vi "Load Offline Map.vi"() -> ()   [LabVIEW 2014]
uses:
  C:/Robotic_Systems/Products/Surveyor/Software/Ground Station/Data/Mapping DLL/GMap.NET.WindowsForms.dll
  Data/Mapping DLL/GMap.NET.WindowsForms.dll
  <vilib>/Utility/miscctls.llb/LVPoint32TypeDef.ctl
  <vilib>/Utility/miscctls.llb/LVPositionTypeDef.ctl
  C:/Robotic_Systems/Products/Surveyor/Software/Ground Station/Data/Mapping DLL/GMap.NET.Core.dll
  Data/Mapping DLL/GMap.NET.Core.dll
  System.Drawing
  System.Windows.Forms
panel:
  in  "Position":T1
  in  "reference out":refnum<k24>
  out "Coords":T2
  out "Lng":dbl format="%#.7g"
  out "Lat":dbl format="%#.7g"
  out "Y":i32
  out "X":i32
  out "Name":string
  out "Case Test":bool
  out "ImportFromGMDB":bool
  in  "Home Button":bool
  out "Center Map Long":dbl format="%#.7g"
  out "Center Map Lat":dbl format="%#.7g"
  out "Current Zoom":dbl
  in  "stop Program":bool
  in  "Offline Map file path (.gmdb)":path
  in  "Map Mode":i32(ring)=2 items=["ServerOnly", "ServerAndCache", "CacheOnly"]
  in  "GMapControl":refnum<k24>(container)
  # "How to Use Map\n\nDragging: hold down right mouse button and move mouse\nZoom: Use mouse scroll Wheel"
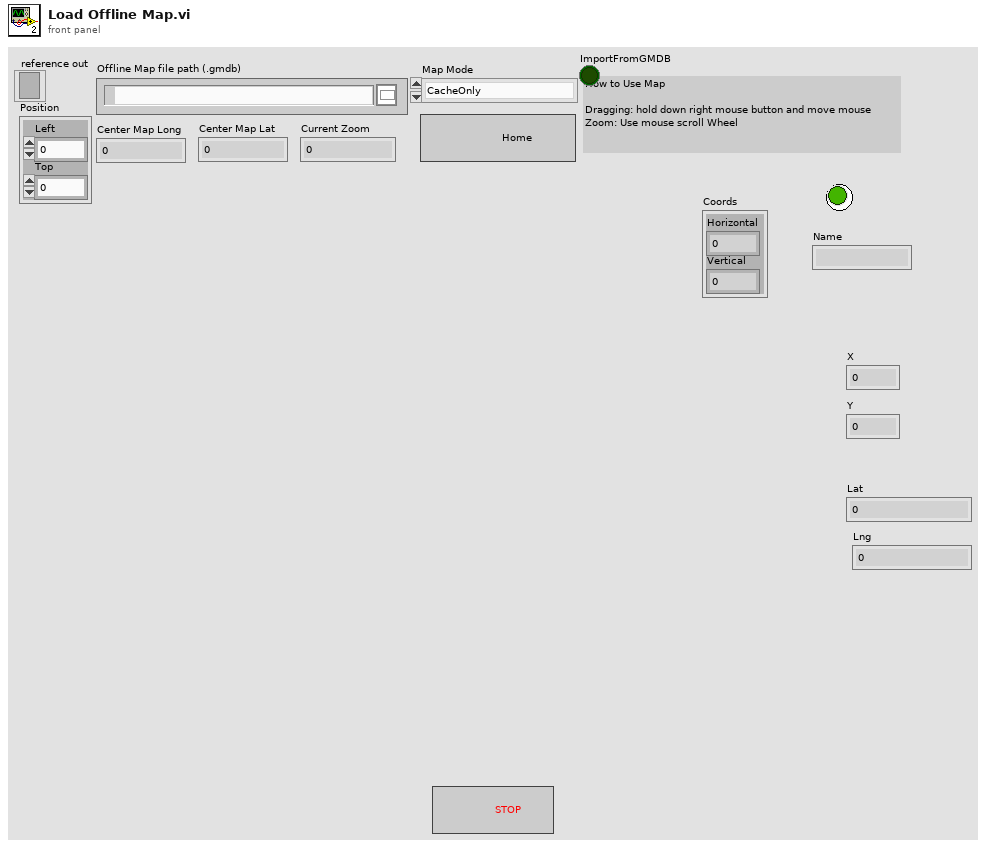
[diagram p1: front panel]
types:
  T1 = typedef "LVPositionTypeDef.ctl" = cluster{"Left":i32, "Top":i32}
  T2 = typedef "LVPoint32TypeDef.ctl" = cluster{"Horizontal":i32, "Vertical":i32}
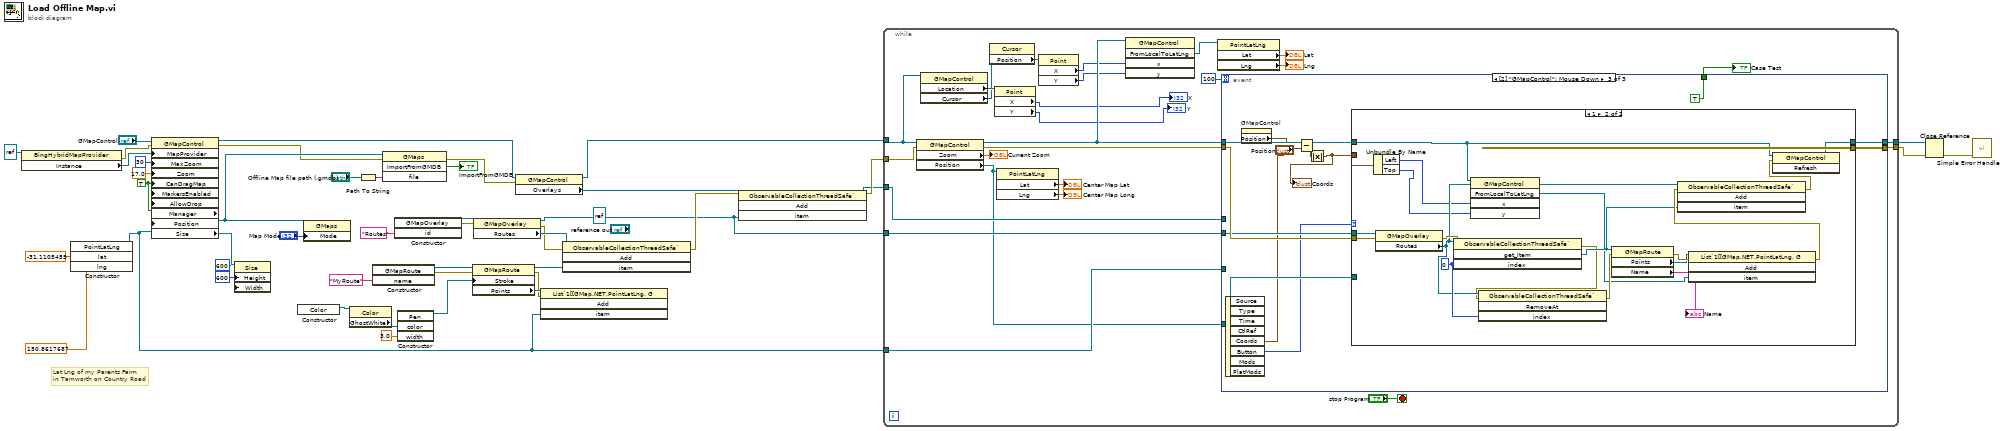
[diagram p0: block diagram]
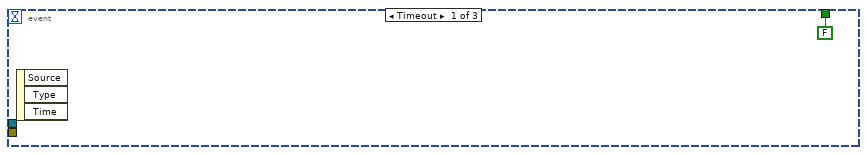
[diagram p2: hidden frame]
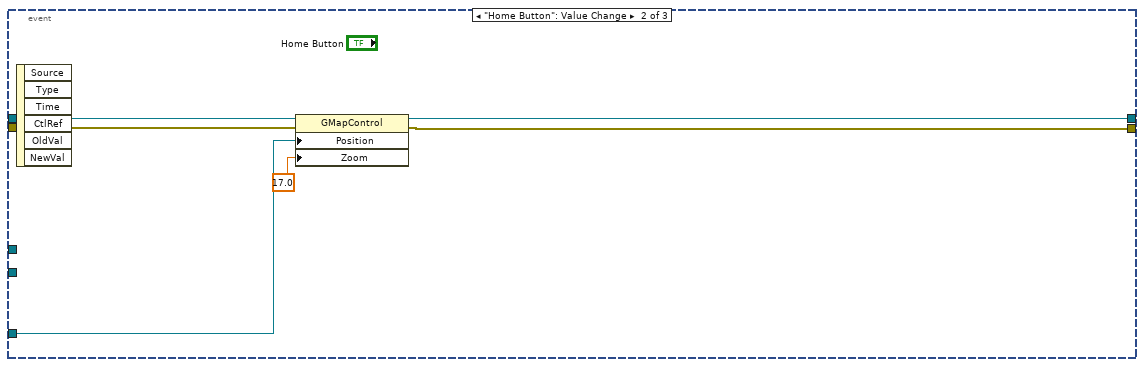
[diagram p3: hidden frame]
diagram:
  (unwired) refnum<k24> refnum ("reference out")
  w41 = TRUE ("CanDragMap")
  # "Lat Lng of my Parents Farm\nin Tamworth on Country Road"
  n1 = property class="BingHybridMapProvider"(reference=refnum<k24> refnum) -> (error out=w33:errorcluster, "Instance"=w43:refnum<k24>)  [unwired: 1 in, 1 out]
  n2 = constructor class="PointLatLng"("lat"=-31.1105459, "lng"=150.8617687) -> (reference out=w9:refnum<k24>)  [unwired: 3 in, 4 out]
  n3 = property class="GMapControl"(reference="GMapControl", error in=w33, "MapProvider"=w43, "MaxZoom"=30, "Zoom"=17.0, "CanDragMap"=w41, "MarkersEnabled"=w41, "AllowDrop"=w41, "Position"=w9) -> (reference out=w24:refnum<k24>, error out=w32:errorcluster, "Manager"=w36:refnum<k24>, "Size"=w3:refnum<k24>)
  n4 = property class="Size"(reference=w3, "Height"=600, "Width"=600) -> ()  [unwired: 1 in, 2 out]
  n5 = constructor class="Color"() -> (reference out=w18:refnum<k24>)  [unwired: 3 in, 2 out]
  n6 = property class="GMaps"(reference=w36, "Mode"="Map Mode") -> ()  [unwired: 1 in, 2 out]
  n7 = property class="Color"(reference=w18) -> ("GhostWhite"=w21:refnum<k24>)  [unwired: 1 in, 2 out]
  n8 = Path To String(path="Offline Map file path (.gmdb)") -> (string=w35:string)
  n9 = constructor class="GMapRoute"("name"="MyRoute") -> (reference out=w5:refnum<k24>, error out=w17:errorcluster)  [unwired: 3 in, 2 out]
  n10 = invoke class="GMaps" method="ImportFromGMDB"(reference=w36, error in=w32, "file"=w35) -> (error out=w25:errorcluster, "ImportFromGMDB"=→"ImportFromGMDB":bool)  [unwired: 1 in, 2 out]
  n11 = constructor class="GMapOverlay"("id"="Routes") -> (reference out=w16:refnum<k24>, error out=w15:errorcluster)  [unwired: 3 in, 2 out]
  n12 = constructor class="Pen"("color"=w21, "width"=sgl 3.0 ("Width")) -> (reference out=w19:refnum<k24>)  [unwired: 3 in, 4 out]
  n13 = property class="GMapRoute"(reference=w5, error in=w17, "Stroke"=w19) -> (reference out=w12:refnum<k24>, error out=w10:errorcluster, "Points"=w11:refnum<k24>)
  n14 = property class="GMapOverlay"(reference=w16, error in=w15) -> (reference out=w6:refnum<k24>, error out=w13:errorcluster, "Routes"=w14:refnum<k24>)
  n15 = property class="GMapControl"(reference=w24, error in=w25) -> (reference out=w8:refnum<k24>, "Overlays"=w27:refnum<k24>)  [unwired: 1 out]
  n16 = invoke class="List`1[[GMap.NET.PointLatLng, G" method="Add"(reference=w11, error in=w10, "item"=w9) -> ()  [unwired: 1 in, 4 out]
  n17 = invoke class="ObservableCollectionThreadSafe`" method="Add"(reference=w14, error in=w13, "item"=w12) -> (error out=w7:errorcluster)  [unwired: 1 in, 3 out]
  n18 = invoke class="ObservableCollectionThreadSafe`" method="Add"(reference=w27, error in=w7, "item"=w6) -> (reference out=w22:refnum<k24>, error out=w23:errorcluster)  [unwired: 1 in, 2 out]
  n19 = while {
    tunnel: w8 -> [w62]
    tunnel: w23 -> [w71]
    tunnel: [w65] -> w31
    tunnel: [w64] -> w30
    tunnel: w9 -> [w63]
    tunnel: w22 -> [w60]
    tunnel: w6 -> [w61]
    stop <- "stop Program" stop-if-true
    n20 = property class="GMapControl"(reference=w62, error in=w71) -> (reference out=w53:refnum<k24>, error out=w67:errorcluster, "Zoom"=→"Current Zoom":dbl, "Position"=w59:refnum<k24>)
    n21 = property class="GMapControl"(reference=w62) -> ("Location"=w52:refnum<k24>, "Cursor"=w49:refnum<k24>)  [unwired: 1 in, 2 out]
    n22 = property class="Cursor"(reference=w49) -> ("Position"=w48:refnum<k24>)  [unwired: 1 in, 2 out]
    n23 = property class="Point"(reference=w52) -> ("X"=→"X":i32, "Y"=→"Y":i32)  [unwired: 1 in, 2 out]
    n24 = property class="PointLatLng"(reference=w59) -> ("Lat"=→"Center Map Lat":dbl, "Lng"=→"Center Map Long":dbl)  [unwired: 1 in, 2 out]
    n25 = property class="Point"(reference=w48) -> ("X"=w47:i32, "Y"=w46:i32)  [unwired: 1 in, 2 out]
    n26 = invoke class="GMapControl" method="FromLocalToLatLng"(reference=w53, "x"=w47, "y"=w46) -> ("FromLocalToLatLng"=w56:refnum<k24>)  [unwired: 2 in, 4 out]
    n27 = property class="PointLatLng"(reference=w56) -> ("Lat"=→"Lat":dbl, "Lng"=→"Lng":dbl)  [unwired: 1 in, 2 out]
    n28 = event shown="[2] \"GMapControl\": Mouse Down" {
      selector: _ -> [_ _ _]
      dyn-events: _ -> [_ _ _]
      timeout: 100 -> [_ _ _]
      tunnel: w53 -> [_ w76 w85]
      tunnel: w67 -> [_ w75 w90]
      tunnel: [_ w78 w87] -> w65
      tunnel: [_ w77 w86] -> w64
      tunnel: w63 -> [_ w74 _]
      tunnel: w61 -> [_ _ w84]
      tunnel: w60 -> [_ _ _]
      tunnel: w59 -> [_ _ w89]
      tunnel: [FALSE ("Case Test") _ TRUE ("Case Test")] -> w57
      event Timeout {
        n29 = event-data() -> ()  [unwired: 1 in, 3 out]
      }
      event "Home Button": Value Change {
        n30 = event-data() -> ()  [unwired: 1 in, 6 out]
        n31 = property class="GMapControl"(reference=w76, error in=w75, "Position"=w74, "Zoom"=17.0) -> (reference out=w78:refnum<k24>, error out=w77:errorcluster)
      }
      event "GMapControl": Mouse Down {
        n32 = event-data() -> ("Coords"=w80:T2, "Button"=w83:u16)  [unwired: 1 in, 6 out]
        n33 = property on="GMapControl" class="AXCont"() -> ("Position"=w82:T1)  [unwired: 2 in, 2 out]
        n34 = Subtract(x=w82, y=w80) -> (x-y=w81:T1)
        n35 = Absolute Value(x=w81) -> (abs(x)=w79:T1)
        "Coords" <- w79
        n36 = case shown="1" w83 {
          tunnel: w90 -> [w91 w111]
          tunnel: w89 -> [_ _]
          tunnel: [w92 w108] -> w87
          tunnel: [w91 w107] -> w86
          tunnel: w85 -> [w92 w93]
          tunnel: w84 -> [_ w105]
          tunnel: w79 -> [_ w97]
          frame 0, Default {
          }
          frame 1 {
            w101 = 0 ("index")
            n37 = Unbundle By Name(w97) -> ("Left"=w96:i32, "Top"=w95:i32)
            n38 = property class="GMapOverlay"(reference=w105, error in=w111) -> (error out=w112:errorcluster, "Routes"=w100:refnum<k24>)  [unwired: 1 out]
            n39 = invoke class="ObservableCollectionThreadSafe`" method="get_Item"(reference=w100, error in=w112, "index"=w101) -> (error out=w99:errorcluster, "get_Item"=w102:refnum<k24>)  [unwired: 1 in, 2 out]
            n40 = invoke class="GMapControl" method="FromLocalToLatLng"(reference=w93, "x"=w96, "y"=w95) -> ("FromLocalToLatLng"=w94:refnum<k24>)  [unwired: 2 in, 4 out]
            n41 = invoke class="ObservableCollectionThreadSafe`" method="RemoveAt"(reference=w100, error in=w99, "index"=w101) -> (error out=w98:errorcluster)  [unwired: 1 in, 3 out]
            n42 = property class="GMapRoute"(reference=w102, error in=w98) -> (error out=w110:errorcluster, "Points"=w106:refnum<k24>, "Name"=→"Name":string)  [unwired: 1 out]
            n43 = invoke class="List`1[[GMap.NET.PointLatLng, G" method="Add"(reference=w106, error in=w110, "item"=w94) -> (error out=w104:errorcluster)  [unwired: 1 in, 3 out]
            n44 = invoke class="ObservableCollectionThreadSafe`" method="Add"(reference=w100, error in=w104, "item"=w102) -> (error out=w103:errorcluster)  [unwired: 1 in, 3 out]
            n45 = invoke class="GMapControl" method="Refresh"(reference=w93, error in=w103) -> (reference out=w108:refnum<k24>, error out=w107:errorcluster)  [unwired: 1 in, 1 out]
          }
        }
      }
    }
    "Case Test" <- w57
  }
  n46 = Close Reference(reference=w31, error in (no error)=w30) -> (error out=w29:errorcluster)
  n47 = call <vilib>:"Simple Error Handler.vi"("error in (no error)"=w29) -> ()  [unwired: 4 in, 5 out]
